vi "test data states.vi"() -> ()   [LabVIEW 2020]
uses:
  configData/configData.lvclass
  C:/Projects/LVOS/EngineeringOS/source/interfaces/data/data.lvclass
  interfaces/data/data.lvclass
  dependencyData/dependencyData.lvclass/dependencyData.ctl
  configData/configData.lvclass/configData.ctl
  dependencyData/dependencyData.lvclass
  C:/Projects/LVOS/EngineeringOS/source/configData/configData.lvclass
  C:/Projects/LVOS/EngineeringOS/source/dependencyData/dependencyData.lvclass
panel:
  out "Boolean":bool
  out "Numeric 2":dbl
  out "Numeric":dbl
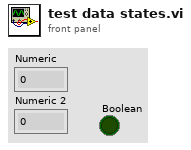
[diagram p1: front panel]
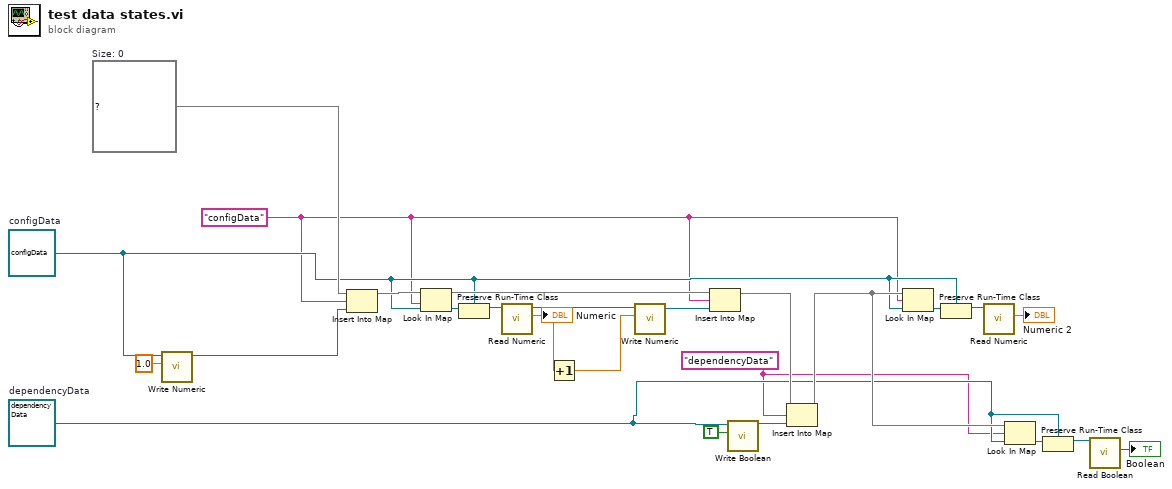
[diagram p0: block diagram]
diagram:
  w1 = "dependencyData"
  w2 = "configData"
  w23 = map{string, refnum<class "data.lvclass">} {}  # Size: 0
  w3 = refnum<class "dependencyData.lvclass"> refnum  # dependencyData
  w4 = refnum<class "configData.lvclass"> refnum  # configData
  n1 = call "Write Numeric.vi"("Numeric"=1.0, "configData in"=w4) -> ("configData out"=w5:refnum<class "configData.lvclass">)  [unwired: 8 in, 1 out]
  n2 = Insert Into Map(map in=w23, key=w2, value=w5) -> (map out=w17:map{string, refnum<class "data.lvclass">})  [unwired: 2 out]
  n3 = Look In Map(map=w17, key=w2, default value=w4) -> (value=w22:refnum<class "data.lvclass">)  [unwired: 1 out]
  n4 = Preserve Run-Time Class(object in=w22, 2:w4) -> (object out=w21:refnum<class "configData.lvclass">)  [unwired: 1 in, 1 out]
  n5 = call "Read Numeric.vi"("configData in"=w21) -> ("Numeric"=w20:dbl, "configData out"=w18:refnum<class "configData.lvclass">)  [unwired: 8 in, 1 out]
  "Numeric" <- w20
  n6 = Increment(x=w20) -> (x+1=w19:dbl)
  n7 = call "Write Numeric.vi"("Numeric"=w19, "configData in"=w18) -> ("configData out"=w16:refnum<class "configData.lvclass">)  [unwired: 8 in, 1 out]
  n8 = Insert Into Map(map in=w17, key=w2, value=w16) -> (map out=w12:map{string, refnum<class "data.lvclass">})  [unwired: 2 out]
  n9 = call "Write Boolean.vi"("Boolean"=TRUE, "dependencyData in"=w3) -> ("dependencyData out"=w11:refnum<class "dependencyData.lvclass">)  [unwired: 8 in, 1 out]
  n10 = Insert Into Map(map in=w12, key=w1, value=w11) -> (map out=w8:map{string, refnum<class "data.lvclass">})  [unwired: 2 out]
  n11 = Look In Map(map=w8, key=w2, default value=w4) -> (value=w14:refnum<class "data.lvclass">)  [unwired: 1 out]
  n12 = Preserve Run-Time Class(object in=w14, 2:w4) -> (object out=w15:refnum<class "configData.lvclass">)  [unwired: 1 in, 1 out]
  n13 = call "Read Numeric.vi"("configData in"=w15) -> ("Numeric"=→"Numeric 2":dbl)  [unwired: 8 in, 2 out]
  n14 = Look In Map(map=w8, key=w1, default value=w3) -> (value=w9:refnum<class "data.lvclass">)  [unwired: 1 out]
  n15 = Preserve Run-Time Class(object in=w9, 2:w3) -> (object out=w7:refnum<class "dependencyData.lvclass">)  [unwired: 1 in, 1 out]
  n16 = call "Read Boolean.vi"("dependencyData in"=w7) -> ("Boolean"=→"Boolean":bool)  [unwired: 8 in, 2 out]
